vi "DataRead.vi"(11 "段名":string) -> (3 "数据":string[][](array[string]))   [LabVIEW 2020]
uses:
  <vilib>/Utility/config.llb/Read Key (String).vi
  <vilib>/Utility/config.llb/NI_LVConfig.lvlib
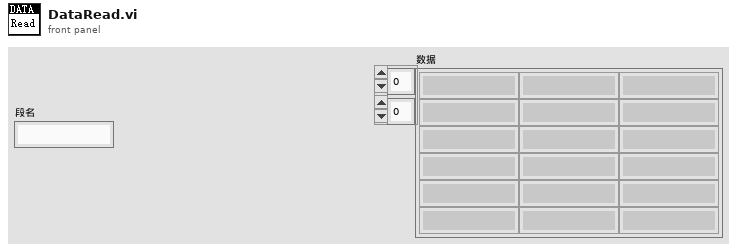
[diagram p1: front panel]
types:
  T1 = typedef "NI_LVConfig.lvlib/Config Data RefNum.ctl" = refnum<k1>
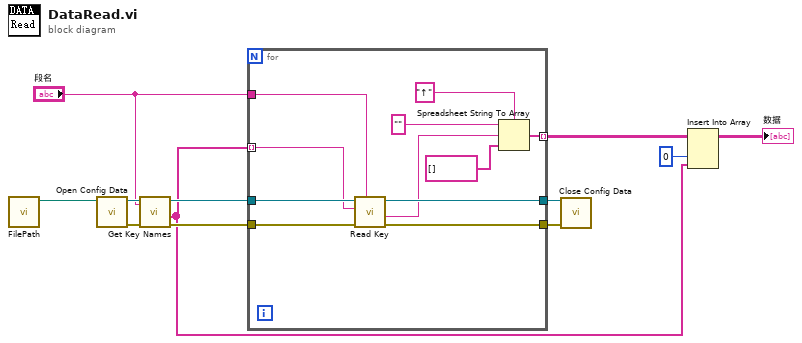
[diagram p0: block diagram]
diagram:
  n1 = call "FilePath.vi"() -> ("添加的路径"=w9:path)  [unwired: 11 in]
  n2 = call <vilib>:"Open Config Data.vi"("configuration file path"=w9) -> ("error out"=w7:errorcluster, "refnum"=w12:T1)  [unwired: 8 in, 1 out]
  n3 = call <vilib>:"Get Key Names.vi"("section"="段名", "error in (no error)"=w7, "refnum"=w12) -> ("error out"=w6:errorcluster, "key names"=w2:string[], "refnum out"=w8:T1)  [unwired: 5 in, 1 out]
  n4 = for {
    tunnel: w2 -> [w20] mode=indexing
    tunnel: "段名" -> [w21]
    tunnel: w8 -> [w23]
    tunnel: w6 -> [w22]
    tunnel: [w19] -> w11
    tunnel: [w18] -> w10
    tunnel: [w14] -> w3 mode=indexing
    n5 = call-poly <vilib>:"Read Key.vi"("section"=w21, "error in (no error)"=w22, "key"=w20, "refnum"=w23) -> ("error out"=w18:errorcluster, "value"=w17:string, "refnum out"=w19:T1)  [unwired: 4 in, 1 out]
    n6 = Spreadsheet String To Array(delimiter (Tab)="↑" ("分隔符(Tab)"), format string="" ("格式字符串"), spreadsheet string=w17, array type (2D Dbl)=string[] []) -> (array=w14:string[])
  }
  n7 = call <vilib>:"Close Config Data.vi"("error in (no error)"=w10, "refnum"=w11) -> ()  [unwired: 8 in, 2 out]
  n8 = Insert Into Array(array=w3, index (col)=0 ("索引 (行)"), new element=w2) -> (→"数据":string[][])  [unwired: 1 in]
